vi "Constructor.vi"(10 "Capacity 2^n":u32) -> (3 "ErrorLog":refnum<class "ErrorLogBuffer.lvclass">)   [LabVIEW 2024, in "ErrorLogBuffer.lvclass"]
uses:
  ErrorLogBuffer.lvclass
  ErrorLogBuffer.lvclass/ErrorLogBuffer.ctl
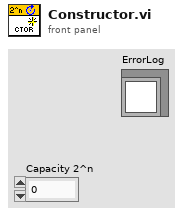
[diagram p1: front panel]
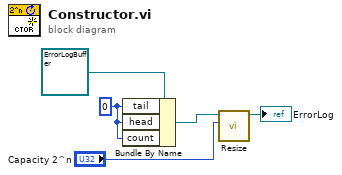
[diagram p0: block diagram]
diagram:
  w1 = 0 ("size")
  n1 = Bundle By Name(cluster=refnum<class "ErrorLogBuffer.lvclass"> refnum ("TypedCircularBuffer.lvclass"), "tail"=w1, "head"=w1, "count"=w1) -> (w4:refnum<class "ErrorLogBuffer.lvclass">)
  n2 = call "Resize.vi"("Capacity 2^n"="Capacity 2^n", "POTTypedCircularBuffer in"=w4) -> ("POTTypedCircularBuffer out"=→"ErrorLog":refnum<class "ErrorLogBuffer.lvclass">)  [unwired: 9 in]
